vi "String.Build Delimited List.vi"(5 "Delimiter":string=", ", 10 "New Data":string, 11 "Existing Str":string) -> (3 "New Str":string)   [LabVIEW 2018]
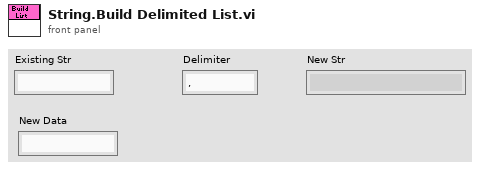
[diagram p1: front panel]
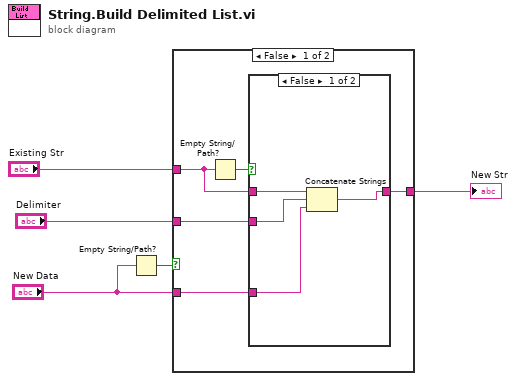
[diagram p0: block diagram]
diagram:
  n1 = Empty String/Path?(string/path="New Data") -> (empty?=w1:bool)
  n2 = case shown="False" w1 {
    tunnel: "Existing Str" -> [w9 w16]
    tunnel: "New Data" -> [w8 _]
    tunnel: "Delimiter" -> [w7 _]
    tunnel: [w6 w16] -> w3
    frame False {
      n3 = Empty String/Path?(string/path=w9) -> (empty?=w10:bool)
      n4 = case shown="False" w10 {
        tunnel: w9 -> [w14 _]
        tunnel: w8 -> [w13 w15]
        tunnel: w7 -> [w12 _]
        tunnel: [w11 w15] -> w6
        frame False {
          n5 = Concatenate Strings(w14, w12, w13) -> (w11:string)
        }
        frame True {
        }
      }
    }
    frame True {
    }
  }
  "New Str" <- w3
